vi "c_ctre_phoenix6_RequestControlDiff_VelocityVoltage_Open.vi"(0 "Numeric 22":u8, 1 "Numeric 2":u32, 2 "Numeric 3":dbl, 3 "Numeric 4":dbl, 4 "Numeric 5":dbl, 5 "Numeric 6":u8, 6 "Numeric 7":dbl, 7 "Numeric 8":i32, 8 "Numeric 9":u8, 9 "Numeric 10":u8, 10 "Numeric 11":u8, 11 "Numeric 12":u8, 12 "Numeric 13":u8, 13 "Numeric 14":u8, 14 "Numeric 15":dbl, 15 "Numeric 16":u8, 16 "Numeric 17":u8, 17 "Numeric 18":u8, 18 "Numeric 19":u8, 19 "Numeric 20":u8) -> (20 "Numeric":i32, 21 "String":string)   [LabVIEW 2025]
uses:
  <vilib>/Rock Robotics/WPI/ThirdParty/Phoenix-LabVIEW/Controls/DriverLib.ctl
panel:
  in  "Numeric 21":u8
  in  "String 2":string
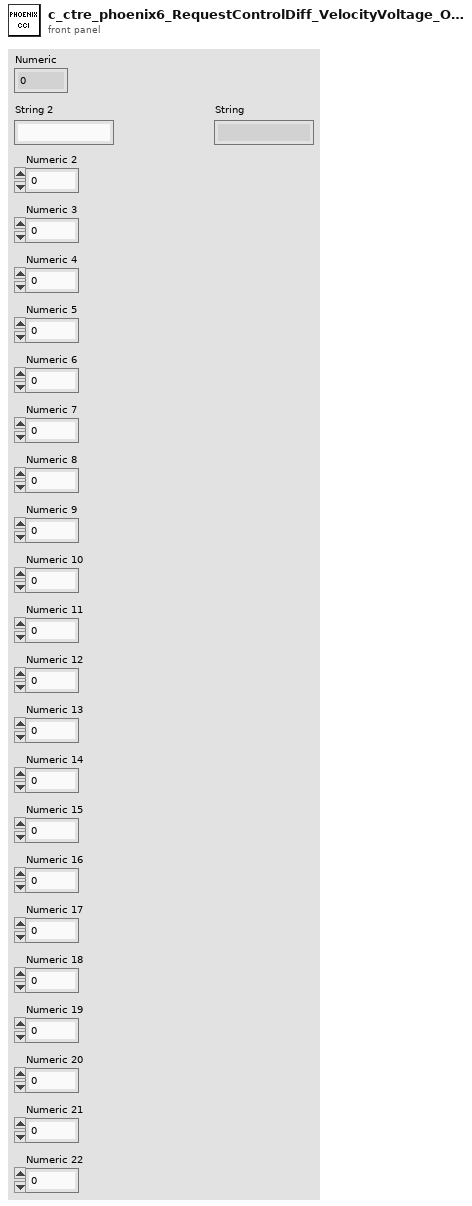
[diagram p1: front panel]
types:
  T1 = typedef "DriverLib.ctl" = path
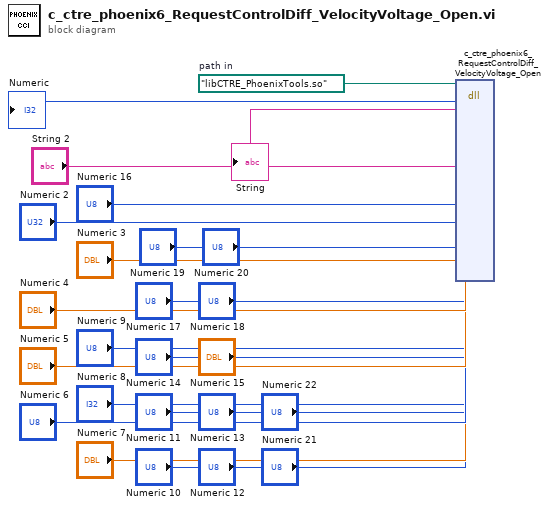
[diagram p0: block diagram]
diagram:
  w25 = T1 path "libCTRE_PhoenixTools.so"  # path in
  n1 = dll-call lib="?" fn="c_ctre_phoenix6_RequestControlDiff_VelocityVoltage_Open"(path in=w25, "String 2", "Numeric 2", "Numeric 3", "Numeric 4", "Numeric 5", "Numeric 6", "Numeric 7", "Numeric 8", "Numeric 9", "Numeric 10", "Numeric 11", "Numeric 12", "Numeric 13", "Numeric 14", "Numeric 15", "Numeric 16", "Numeric 17", "Numeric 18", "Numeric 19", "Numeric 20", "Numeric 21", "Numeric 22") -> (→"Numeric":i32, →"String":string)  [unwired: 23 in, 2 out]
